vi "4th_PWM_Control.vi"(8 "error in":errorcluster, 10 "PWM":cluster{"Frequence":dbl, "DutyCycle":dbl}, 11 "Motor_Type":T1) -> (0 "error out":errorcluster)   [LabVIEW 2019]
uses:
  Motor_Type.ctl
  <vilib>/Utility/error.llb/Error Cluster From Error Code.vi
  <vilib>/rvi/errors/niLvFpgaAdjustHostInterfaceError.vi
  <vilib>/rvi/interface/nirviReadWriteControl/nirviReadWriteControl.xnode
  NiFpgaLv.dll
  <vilib>/rvi/interface/Simulation/niFpgaSimulationCallBeginRW.vi
  KNRm_ReMi_OS6_436Motor.lvlibp
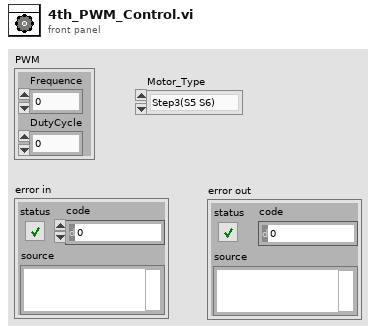
[diagram p1: front panel]
types:
  T1 = typedef "Motor_Type.ctl" = enum16{"Step3(S5 S6)", "Step2(S3 S4)", "Step1(S1 S2)"}
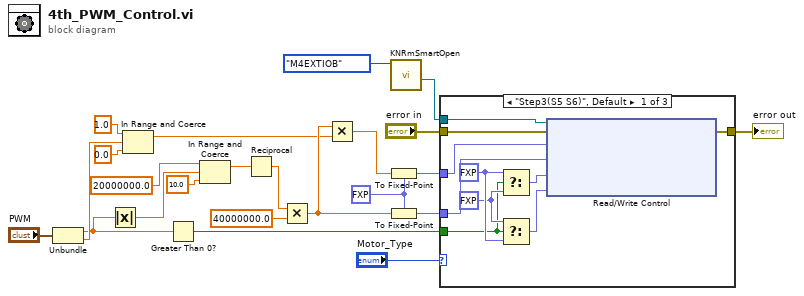
[diagram p0: block diagram]
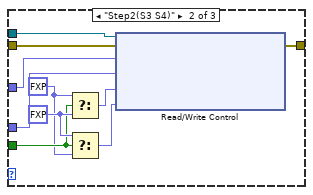
[diagram p2: hidden frame]
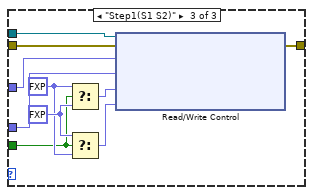
[diagram p3: hidden frame]
diagram:
  w17 = fxp<+,22,22> 0.0 ("fixed-point")
  n1 = Unbundle("PWM") -> ("Frequence"=w3:dbl, "DutyCycle"=w21:dbl)
  n2 = Absolute Value(x=w3) -> (abs(x)=w4:dbl)
  n3 = In Range and Coerce(upper limit=1.0, x=w21, lower limit=0.0) -> (coerced(x)=w20:dbl)  [unwired: 1 out]
  n4 = Greater Than 0?(x=w3) -> (x > 0?=w5:bool)
  n5 = In Range and Coerce(upper limit=20000000.0, x=w4, lower limit=10.0) -> (coerced(x)=w18:dbl)  [unwired: 1 out]
  n6 = Reciprocal(x=w18) -> (1/x=w19:dbl)
  n7 = Multiply(x=w19, y=40000000.0) -> (x*y=w22:dbl)
  n8 = Multiply(x=w22, y=w20) -> (x*y=w23:dbl)
  n9 = To Fixed-Point(fixed-point type=w17, number=w23) -> (fixed-point=w11:fxp<+,22,22>)
  n10 = To Fixed-Point(fixed-point type=w17, number=w22) -> (fixed-point=w9:fxp<+,22,22>)
  n11 = call "KNRmSmartOpen.vi"("INI FPGA MODE"=enum16{"Original", "M4EXTIOB"}."M4EXTIOB") -> ("FPGA VI Reference for EXTIOB"=w1:refnum<k20>)  [unwired: 7 in, 3 out]
  n12 = case shown="\"Step3(S5 S6)\", Default" "Motor_Type" {
    tunnel: w9 -> [w33 w41 w51]
    tunnel: w11 -> [w32 w42 w52]
    tunnel: w1 -> [w31 w43 w53]
    tunnel: [w30 w40 w50] -> w8
    tunnel: "error in" -> [w29 w39 w49]
    tunnel: w5 -> [w26 w37 w46]
    frame "Step3(S5 S6)", Default {
      w28 = fxp<+,22,22> 0.0 ("S1(P_HightLevelTime(tick)")
      w27 = fxp<+,22,22> 1.0 ("S1(P_HightLevelTime(tick)")
      n13 = Select(t=w28, s=w26, f=w27) -> (s? t:f=w24:fxp<+,22,22>)
      n14 = Select(t=w27, s=w26, f=w28) -> (s? t:f=w25:fxp<+,22,22>)
      n15 = xnode "Read/Write Control"("FPGA VI Reference In"=w31, "error in"=w29, "S5(P)_HightLevelTime(tick)"=w32, "S5(P)_CycleTime(tick)"=w33, "S6(D)_HightLevelTime(tick)"=w24, "S6(D)_CycleTime(tick)"=w25) -> ("error out"=w30:errorcluster)  [unwired: 1 out]
    }
    frame "Step2(S3 S4)" {
      w36 = fxp<+,22,22> 0.0 ("S1(P_HightLevelTime(tick)")
      w38 = fxp<+,22,22> 1.0 ("S1(P_HightLevelTime(tick)")
      n16 = Select(t=w36, s=w37, f=w38) -> (s? t:f=w34:fxp<+,22,22>)
      n17 = Select(t=w38, s=w37, f=w36) -> (s? t:f=w35:fxp<+,22,22>)
      n18 = xnode "Read/Write Control"("FPGA VI Reference In"=w43, "error in"=w39, "S3(P)_HightLevelTime(tick)"=w42, "S3(P)CycleTime(tick)"=w41, "S4(D)_HightLevelTime(tick)"=w34, "S4(D)_CycleTime(tick)"=w35) -> ("error out"=w40:errorcluster)  [unwired: 1 out]
    }
    frame "Step1(S1 S2)" {
      w47 = fxp<+,22,22> 0.0 ("S1(P_HightLevelTime(tick)")
      w48 = fxp<+,22,22> 1.0 ("S1(P_HightLevelTime(tick)")
      n19 = Select(t=w47, s=w46, f=w48) -> (s? t:f=w45:fxp<+,22,22>)
      n20 = Select(t=w48, s=w46, f=w47) -> (s? t:f=w44:fxp<+,22,22>)
      n21 = xnode "Read/Write Control"("FPGA VI Reference In"=w53, "error in"=w49, "S1(P_HightLevelTime(tick)"=w52, "S1(P)_CycleTime(tick)"=w51, "S2(D)_HightLevelTime(tick)"=w45, "S2(D)_CycleTime(tick)"=w44) -> ("error out"=w50:errorcluster)  [unwired: 1 out]
    }
  }
  "error out" <- w8
